vi "SlideyStop.vi"() -> ()   [LabVIEW 2018]
uses:
  Pane Object.lvclass/Pane Position Enum.ctl
  Boolean Object.lvclass/Boolean Object Position.lvclass
  Pane Object.lvclass/Pane Object Position.lvclass
panel:
  in  "Reverse!":bool
  in  "Stop":bool
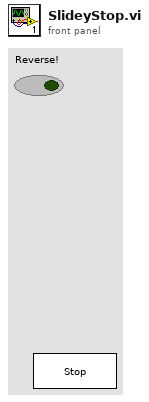
[diagram p1: front panel]
types:
  T1 = typedef "Pane Object Position.lvclass/Pane Position Enum.ctl" = enum16{"Indeterminate", "Top", "Right", "Top Right", "Bottom", "5", "Bottom Right", "7", "Left", "Top Left", "10", "11", "Bottom Left"}
  T2 = typedef "Pane Object Position.lvclass/Object Coordinates.ctl" = cluster{"Top":i32, "Right":i32, "Bottom":i32, "Left":i32}
  T3 = typedef "Direction Ctl.ctl" = enum16{"Right", "Left", "Up", "Down"}
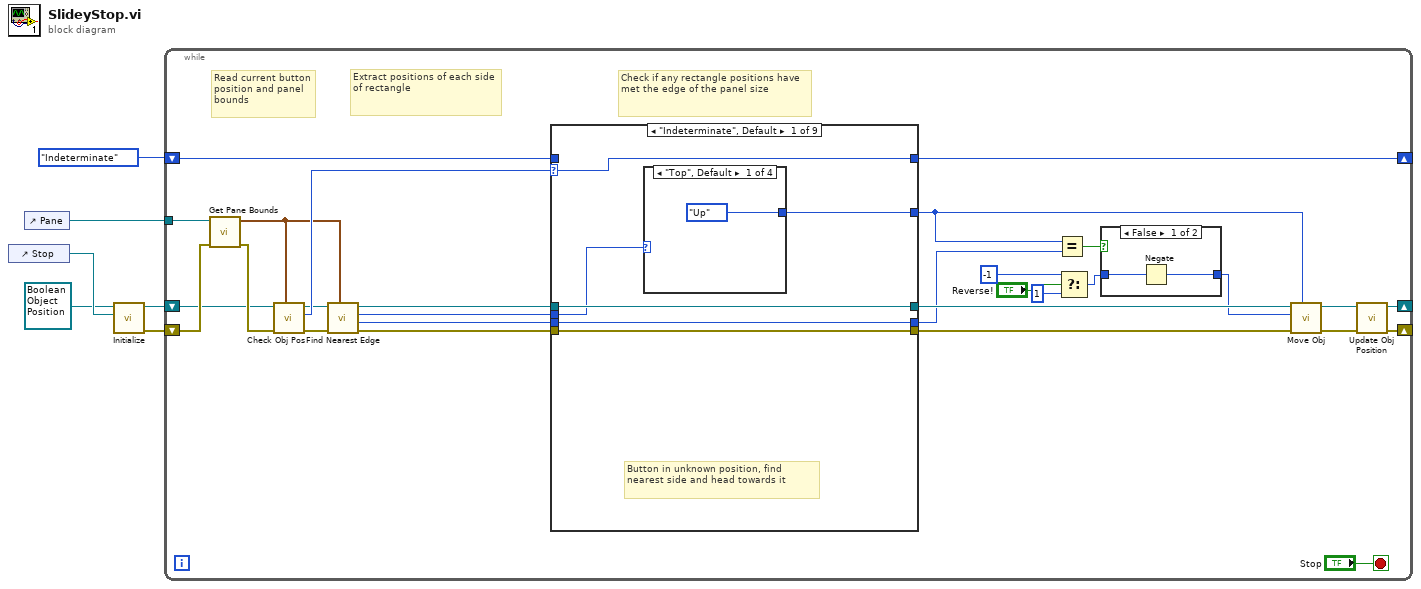
[diagram p0: block diagram]
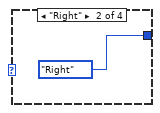
[diagram p2: hidden frame]
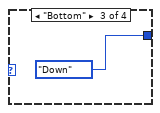
[diagram p3: hidden frame]
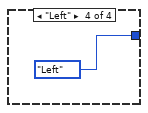
[diagram p4: hidden frame]
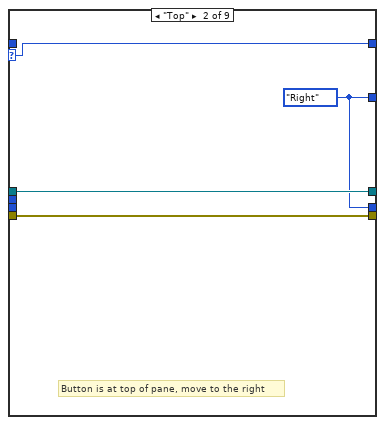
[diagram p5: hidden frame]
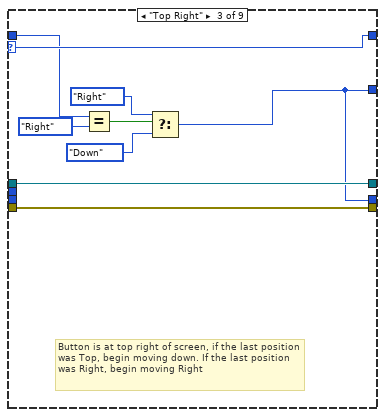
[diagram p6: hidden frame]
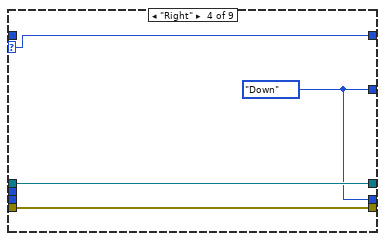
[diagram p7: hidden frame]
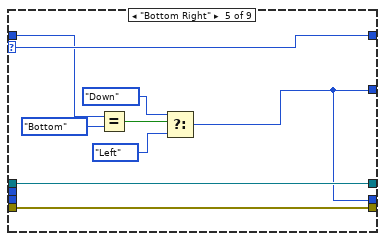
[diagram p8: hidden frame]
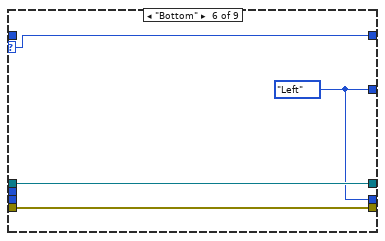
[diagram p9: hidden frame]
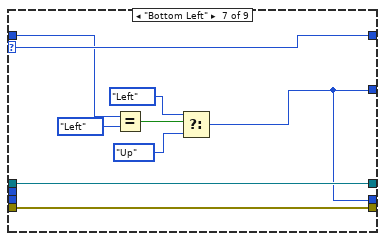
[diagram p10: hidden frame]
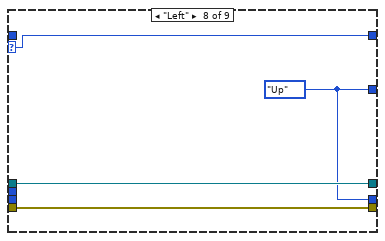
[diagram p11: hidden frame]
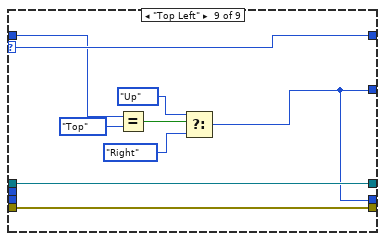
[diagram p12: hidden frame]
diagram:
  n1 = control-ref of="Stop"() -> (w5:refnum<vi>)
  n2 = control-ref of="Pane"() -> (w2:refnum<vi>)
  n3 = call-dynamic "Initialize.vi"("Ctl Refnum"=w5, "Boolean Object Position in"=refnum<class "Boolean Object Position.lvclass"> refnum ("Boolean Object Position.lvclass")) -> ("error out"=w1:errorcluster, "Boolean Object Position out"=w3:refnum<class "Boolean Object Position.lvclass">)  [unwired: 8 in]
  n4 = while {
    shift-right: [w33] -> _
    shift-left: Pane_Position_Enum."Indeterminate" -> [w34]
    tunnel: w2 -> [w32]
    shift-right: [w21] -> _
    shift-left: w1 -> [w31]
    shift-right: [w22] -> _
    shift-left: w3 -> [w29]
    stop <- "Stop" stop-if-true
    # "Check if any rectangle positions have met the edge of the panel size"
    # "Extract positions of each side of rectangle"
    # "Read current button position and panel bounds"
    n5 = call "Get Pane Bounds.vi"("error in (no error)"=w31, "Pane"=w32) -> ("error out"=w30:errorcluster, "Panel Coordinates"=w17:T2)  [unwired: 8 in]
    n6 = call-dynamic "Check Obj Pos.vi"("Pane Coordinates"=w17, "error in (no error)"=w30, "Boolean Object Position in"=w29) -> ("error out"=w27:errorcluster, "Position"=w28:T1, "Boolean Object Position out"=w19:refnum<class "Boolean Object Position.lvclass">)  [unwired: 6 in]
    n7 = call-dynamic "Find Nearest Edge.vi"("Pane Coordinates"=w17, "error in (no error)"=w27, "Boolean Object Position in"=w19) -> ("error out"=w20:errorcluster, "Direction"=w15:T3, "Nearest Side"=w16:T1, "Boolean Object Position out"=w18:refnum<class "Boolean Object Position.lvclass">)  [unwired: 5 in]
    n8 = case shown="\"Indeterminate\", Default" w28 {
      selector: w28 -> [w40 w47 w52 w60 w69 w73 w82 w86 w95]
      tunnel: w34 -> [_ _ w51 _ w64 _ w77 _ w90]
      tunnel: [w40 w47 w52 w60 w69 w73 w82 w86 w95] -> w33
      tunnel: w18 -> [w39 w49 w58 w62 w71 w75 w84 w88 w97]
      tunnel: w20 -> [w38 w48 w57 w61 w70 w74 w83 w87 w96]
      tunnel: [w39 w49 w58 w62 w71 w75 w84 w88 w97] -> w26
      tunnel: [w38 w48 w57 w61 w70 w74 w83 w87 w96] -> w25
      tunnel: [w41 w46 w50 w59 w63 w72 w76 w85 w89] -> w13
      tunnel: w16 -> [w37 _ _ _ _ _ _ _ _]
      tunnel: w15 -> [w36 _ _ _ _ _ _ _ _]
      tunnel: [w36 w46 w50 w59 w63 w72 w76 w85 w89] -> w12
      frame "Indeterminate", Default {
        # "Button in unknown position, find nearest side and head towards it"
        n9 = case shown="\"Top\", Default" w37 {
          tunnel: [enum16{"Right", "Left", "Up", "Down"}."Up" ("Direction") enum16{"Right", "Left", "Up", "Down"}."Right" ("Direction") enum16{"Right", "Left", "Up", "Down"}."Down" ("Direction") enum16{"Right", "Left", "Up", "Down"}."Left" ("Direction")] -> w41
          frame "Top", Default {
          }
          frame "Right" {
          }
          frame "Bottom" {
          }
          frame "Left" {
          }
        }
      }
      frame "Top" {
        w46 = enum16{"Right", "Left", "Up", "Down"}."Right" ("Direction")
        # "Button is at top of pane, move to the right"
      }
      frame "Top Right" {
        # "Button is at top right of screen, if the last position was Top, begin moving down. If the last position was Right, begin moving Right"
        n10 = Equal?(x=w51, y=Pane_Position_Enum."Right") -> (x = y?=w55:bool)
        n11 = Select(t=enum16{"Right", "Left", "Up", "Down"}."Right" ("Direction"), s=w55, f=enum16{"Right", "Left", "Up", "Down"}."Down") -> (s? t:f=w50:enum16{"Right", "Left", "Up", "Down"})
      }
      frame "Right" {
        w59 = enum16{"Right", "Left", "Up", "Down"}."Down" ("Direction")
      }
      frame "Bottom Right" {
        n12 = Equal?(x=w64, y=Pane_Position_Enum."Bottom") -> (x = y?=w67:bool)
        n13 = Select(t=enum16{"Right", "Left", "Up", "Down"}."Down" ("Direction"), s=w67, f=enum16{"Right", "Left", "Up", "Down"}."Left") -> (s? t:f=w63:enum16{"Right", "Left", "Up", "Down"})
      }
      frame "Bottom" {
        w72 = enum16{"Right", "Left", "Up", "Down"}."Left" ("Direction")
      }
      frame "Bottom Left" {
        n14 = Equal?(x=w77, y=Pane_Position_Enum."Left") -> (x = y?=w80:bool)
        n15 = Select(t=enum16{"Right", "Left", "Up", "Down"}."Left" ("Direction"), s=w80, f=enum16{"Right", "Left", "Up", "Down"}."Up") -> (s? t:f=w76:enum16{"Right", "Left", "Up", "Down"})
      }
      frame "Left" {
        w85 = enum16{"Right", "Left", "Up", "Down"}."Up" ("Direction")
      }
      frame "Top Left" {
        n16 = Equal?(x=w90, y=Pane_Position_Enum."Top") -> (x = y?=w93:bool)
        n17 = Select(t=enum16{"Right", "Left", "Up", "Down"}."Up" ("Direction"), s=w93, f=enum16{"Right", "Left", "Up", "Down"}."Right") -> (s? t:f=w89:enum16{"Right", "Left", "Up", "Down"})
      }
    }
    n18 = Equal?(x=w13, y=w12) -> (x = y?=w14:bool)
    n19 = Select(t=-1 ("Speed"), s="Reverse!", f=1) -> (s? t:f=w7:i32)
    n20 = case shown="False" w14 {
      tunnel: w7 -> [w99 w100]
      tunnel: [w98 w100] -> w11
      frame False {
        n21 = Negate(x=w99) -> (-x=w98:i32)
      }
      frame True {
      }
    }
    n22 = call-dynamic "Move Obj.vi"("Direction"=w13, "error in (no error)"=w25, "Magnitude"=w11, "Pane Object Position in"=w26) -> ("error out"=w23:errorcluster, "Pane Object Position out"=w24:refnum<class "Boolean Object Position.lvclass">)  [unwired: 6 in]
    n23 = call-dynamic "Update Obj Position.vi"("error in (no error)"=w23, "Boolean Object Position in"=w24) -> ("error out"=w21:errorcluster, "Boolean Object Position out"=w22:refnum<class "Boolean Object Position.lvclass">)  [unwired: 8 in]
  }
